vi "PH_TraceAndHisto.vi"(0 "Data In":u32[](array[numeric]), 1 "Reset":bool, 5 "Data Count":i32, 11 "Trace Bins":i32=25) -> (4 "Histograms":i32[][](array[numeric]), 6 "Total Photon Count":u64[](array[numeric]), 13 "Total Oveflow Count":u64, 14 "Num Records Total":i32, 15 "Traces":i32[][](array[numeric]))   [LabVIEW 2010]
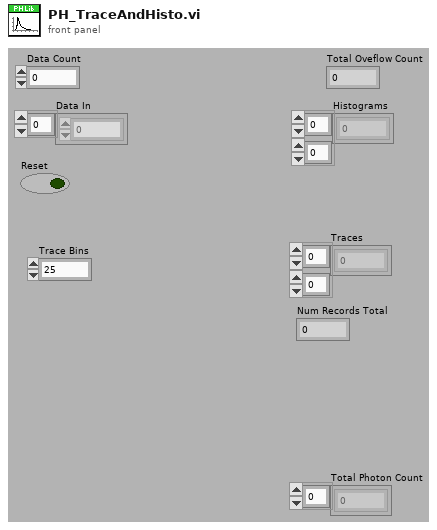
[diagram p1: front panel]
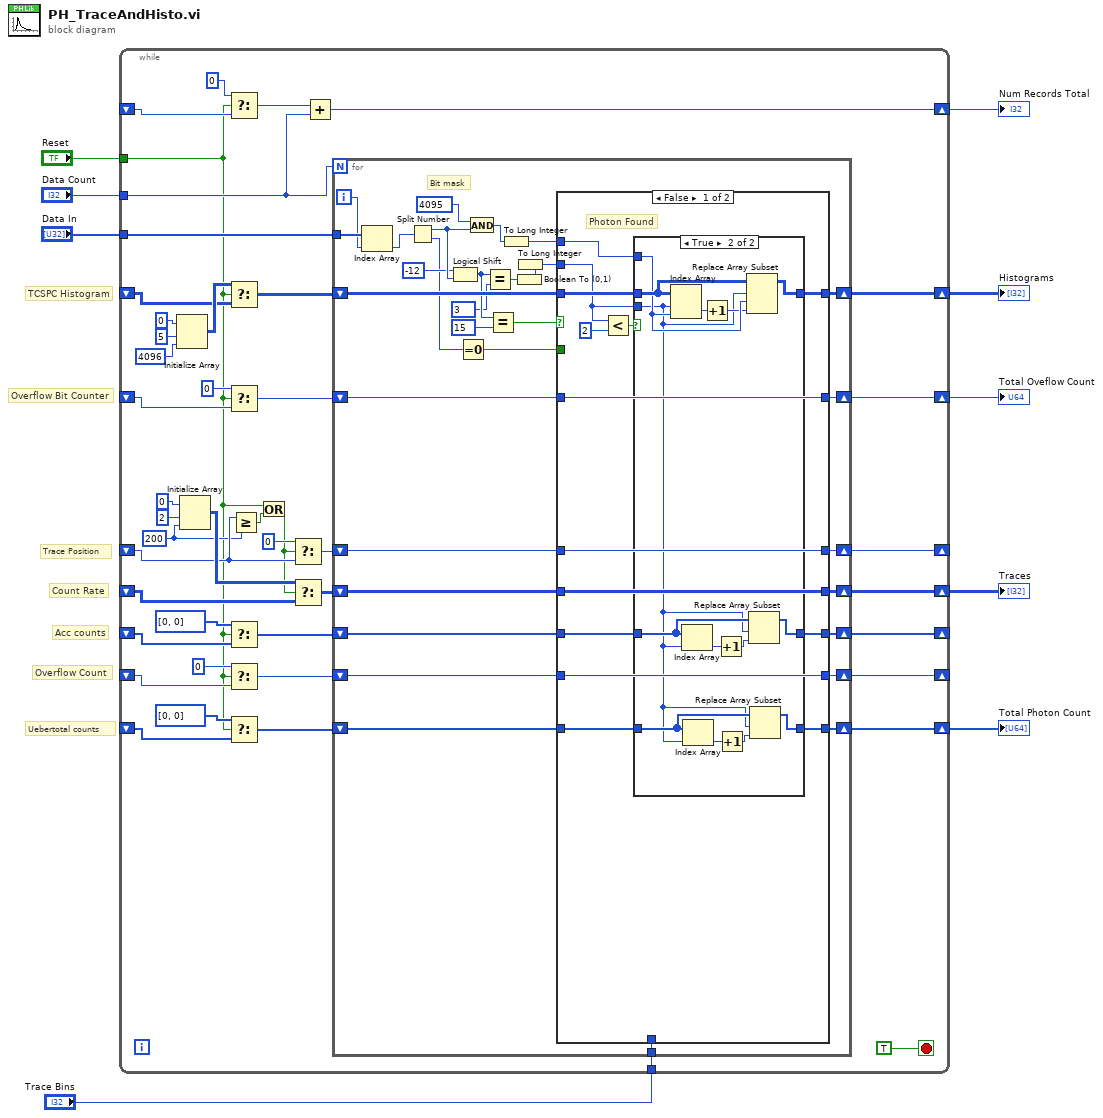
[diagram p0: block diagram]
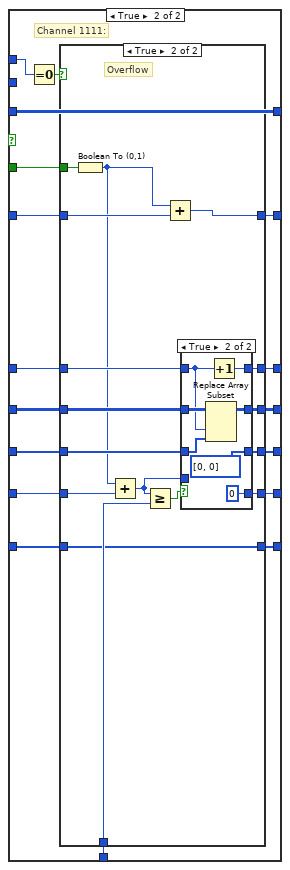
[diagram p3: hidden frame]
diagram:
  # "Uebertotal counts"
  # "Trace Position"
  # "Overflow Count"
  # "Acc counts"
  # "Count Rate"
  # "TCSPC Histogram"
  # "Overflow Bit Counter"
  n1 = while {
    tunnel: "Data In" -> [w52]
    shift-right: [w53] -> w9
    shift-left: _ -> [w48]
    tunnel: "Reset" -> [w10]
    shift-right: [w45] -> w2
    shift-left: _ -> [w44]
    shift-right: [w40] -> w5
    shift-left: _ -> [w39]
    shift-right: [w37] -> _
    shift-left: _ -> [w36]
    shift-right: [w34] -> _
    shift-left: _ -> [w33]
    tunnel: "Trace Bins" -> [w32]
    shift-right: [w29] -> _
    shift-left: _ -> [w27]
    tunnel: "Data Count" -> [w22]
    shift-right: [w21] -> w3
    shift-left: _ -> [w24]
    shift-right: [w12] -> w1
    shift-left: _ -> [w11]
    stop <- TRUE stop-if-true
    w18 = 200 ("dimension size")
    n2 = Initialize Array(0 ("element"), 5 ("dimension size"), 4096 ("dimension size")) -> (w49:i32[][])
    n3 = Initialize Array(0 ("element"), 2 ("dimension size"), w18) -> (w42:i32[][])
    n4 = Select(t=0 ("Data Count 2"), s=w10, f=w24) -> (s? t:f=w23:i32)
    n5 = Select(t=w49, s=w10, f=w48) -> (s? t:f=w50:i32[][])
    n6 = Select(t=u64 0, s=w10, f=w44) -> (s? t:f=w46:u64)
    n7 = Select(t=u32[] [0, 0] ("initialized array"), s=w10, f=w36) -> (s? t:f=w38:u32[])
    n8 = Select(t=u32 0, s=w10, f=w33) -> (s? t:f=w35:u32)
    n9 = Select(t=u64[] [0, 0] ("initialized array"), s=w10, f=w11) -> (s? t:f=w13:u64[])
    n10 = Greater Or Equal?(x=w27, y=w18) -> (x >= y?=w28:bool)
    n11 = Or(x=w10, y=w28) -> (x .or. y?=w26:bool)
    n12 = Select(t=0, s=w26, f=w27) -> (s? t:f=w30:i32)
    n13 = Select(t=w42, s=w26, f=w39) -> (s? t:f=w41:i32[][])
    n14 = Add(x=w23, y=w22) -> (x+y=w21:i32)
    n15 = for {
      N: w22 -> [_]
      tunnel: w52 -> [w64]
      shift-right: [w82] -> w53
      shift-left: w50 -> [w84]
      shift-right: [w76] -> w45
      shift-left: w46 -> [w77]
      shift-right: [w71] -> w40
      shift-left: w41 -> [w72]
      shift-right: [w73] -> w37
      shift-left: w38 -> [w74]
      shift-right: [w69] -> w34
      shift-left: w35 -> [w70]
      tunnel: w32 -> [w68]
      shift-right: [w66] -> w29
      shift-left: w30 -> [w67]
      shift-right: [w55] -> w12
      shift-left: w13 -> [w56]
      i -> [w63]
      # "Bit mask"
      n16 = Index Array(array=w64, index=w63) -> (element=w62:u32)
      n17 = Split Number(x=w62) -> (hi(x)=w81:u16, lo(x)=w65:u16)
      n18 = Logical Shift(y=i8 -12, x=w81) -> (x << y=w61:u16)
      n19 = Equal To 0?(x=w65) -> (x = 0?=w75:bool)
      n20 = And(x=u16 4095, y=w81) -> (x .and. y?=w85:u16)
      n21 = Equal?(x=w61, y=u16 3) -> (x = y?=w59:bool)
      n22 = Equal?(x=w61, y=u16 15) -> (x = y?=w78:bool)
      n23 = To Long Integer(number=w85) -> (32bit integer=w83:i32)
      n24 = Boolean To (0,1)(Boolean=w59) -> (0, 1=w58:i16)
      n25 = To Long Integer(number=w58) -> (32bit integer=w57:i32)
      n26 = case shown="False" w78 {
        tunnel: w84 -> [w100 w131]
        tunnel: w83 -> [w94 w120]
        tunnel: [w99 w131] -> w82
        tunnel: w57 -> [w90 _]
        tunnel: w77 -> [w98 w133]
        tunnel: [w98 w132] -> w76
        tunnel: w75 -> [_ w130]
        tunnel: w74 -> [w93 w128]
        tunnel: [w92 w124] -> w73
        tunnel: w72 -> [w97 w127]
        tunnel: [w97 w123] -> w71
        tunnel: w70 -> [w96 w129]
        tunnel: [w96 w125] -> w69
        tunnel: w68 -> [_ w126]
        tunnel: w67 -> [w95 w122]
        tunnel: [w95 w121] -> w66
        tunnel: w56 -> [w88 w119]
        tunnel: [w87 w118] -> w55
        frame False {
          # "Photon Found"
          n27 = Less?(x=w90, y=2) -> (x < y?=w91:bool)
          n28 = case shown="True" w91 {
            tunnel: w100 -> [w103 w117]
            tunnel: [w103 w116] -> w99
            tunnel: w94 -> [_ w115]
            tunnel: w90 -> [_ w104]
            tunnel: w93 -> [w102 w114]
            tunnel: [w102 w113] -> w92
            tunnel: w88 -> [w101 w106]
            tunnel: [w101 w105] -> w87
            frame False {
            }
            frame True {
              n29 = Index Array(array=w117, index (row)=w104, index (col)=w115) -> (element=w112:i32)
              n30 = Index Array(array=w114, index=w104) -> (element=w110:u32)
              n31 = Index Array(array=w106, index=w104) -> (element=w108:u64)
              n32 = Increment(x=w112) -> (x+1=w111:i32)
              n33 = Increment(x=w110) -> (x+1=w109:u32)
              n34 = Increment(x=w108) -> (x+1=w107:u64)
              n35 = Replace Array Subset(array=w117, new element=w111, index (row)=w104, index (col)=w115) -> (w116:i32[][])
              n36 = Replace Array Subset(array=w114, new element=w109, index=w104) -> (w113:u32[])
              n37 = Replace Array Subset(array=w106, new element=w107, index=w104) -> (w105:u64[])
            }
          }
        }
        frame True {
          # "Channel 1111:"
          n38 = Equal To 0?(x=w120) -> (x = 0?=w134:bool)
          n39 = case shown="True" w134 {
            tunnel: w133 -> [w140 w156]
            tunnel: [w140 w155] -> w132
            tunnel: w130 -> [_ w142]
            tunnel: w129 -> [w139 w145]
            tunnel: w128 -> [w138 w151]
            tunnel: w127 -> [w137 w149]
            tunnel: w126 -> [_ w154]
            tunnel: [w139 w152] -> w125
            tunnel: [w138 w150] -> w124
            tunnel: [w137 w148] -> w123
            tunnel: w122 -> [w136 w147]
            tunnel: [w136 w146] -> w121
            tunnel: w119 -> [w135 w141]
            tunnel: [w135 w141] -> w118
            frame False {
              # "Trigger Signal"
            }
            frame True {
              # "Overflow"
              n40 = Boolean To (0,1)(Boolean=w142) -> (0, 1=w143:i16)
              n41 = Add(x=w143, y=w145) -> (x+y=w144:u32)
              n42 = Greater Or Equal?(x=w144, y=w154) -> (x >= y?=w153:bool)
              n43 = Add(x=w143, y=w156) -> (x+y=w155:u64)
              n44 = case shown="True" w153 {
                tunnel: w144 -> [w160 _]
                tunnel: [w160 u32 0] -> w152
                tunnel: w151 -> [w159 w165]
                tunnel: [w159 u32[] [0, 0] ("initialized array")] -> w150
                tunnel: w149 -> [w158 w166]
                tunnel: [w158 w164] -> w148
                tunnel: w147 -> [w157 w162]
                tunnel: [w157 w163] -> w146
                frame False {
                }
                frame True {
                  n45 = Replace Array Subset(array=w166, new element=w165, index (col)=w162) -> (w164:i32[][])  [unwired: 1 in]
                  n46 = Increment(x=w162) -> (x+1=w163:i32)
                }
              }
            }
          }
        }
      }
    }
  }
  "Histograms" <- w9
  "Traces" <- w5
  "Num Records Total" <- w3
  "Total Oveflow Count" <- w2
  "Total Photon Count" <- w1
